vi "Create from SSH.vi"(8 "Error In":errorcluster, 11 "SSH":refnum<class "SSH.lvclass">) -> (0 "Error Out":errorcluster, 3 "Known Host":refnum<class "Known Host.lvclass">)   [LabVIEW 2018, in "Toolkit.lvlib" / "Known Host.lvclass"]
doc: "Creates a new Known Host object that represents a libssh2lv shared library Known Host struct. This VI must be called, or executed, before using any other Known Host-related VIs. This VI allocates memory within the libssh2lv shared library that must be explicitly deallocated, or freed, at the end of the application using the <B>Destroy</B> VI to avoid memory leaks or running Out-of-Memory (OOM) on a resource contrained system.\n\nA Known Host object represents the read-only data obtained about an entry in a known hosts file on the local host."
uses:
  Known Host.lvclass
  SSH/SSH.lvclass
  SSH/SSH.lvclass/SSH.ctl
  Known Host.lvclass/Known Host.ctl
  Toolkit.lvlib
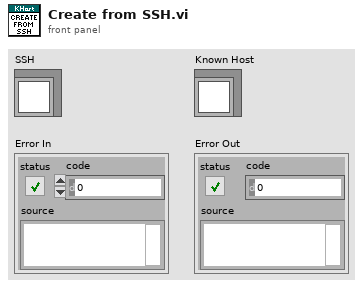
[diagram p1: front panel]
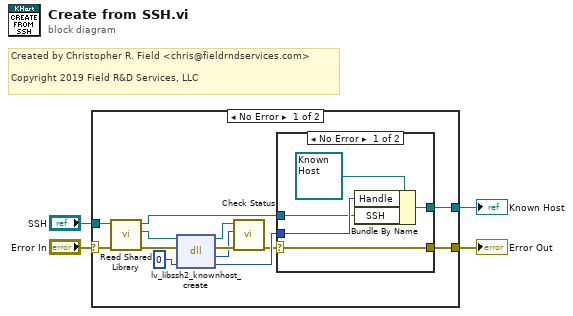
[diagram p0: block diagram]
diagram:
  # "Created by Christopher R. Field <chris@fieldrndservices.com>\n\nCopyright 2019 Field R&D Services, LLC"
  n1 = case shown="No Error" "Error In" {
    selector: "Error In" -> [w8 w24]
    tunnel: [w10 w24] -> w3
    tunnel: [w17 _] -> w2
    tunnel: "SSH" -> [w9 _]
    frame No Error {
      n2 = call "Read Shared Library.vi"("Error In"=w8, "SSH In"=w9) -> ("Error Out"=w7:errorcluster, "libssh2lv Shared Library"=w6:path, "SSH Out"=w5:refnum<class "SSH.lvclass">)  [unwired: 7 in]
      n3 = dll-call lib="D:/Users/cfield/Code/Field R&D Services/SSH/LV-LIBSSH2/LabVIEW/trunk/src/Toolkit/Support/lv-libssh2.*" fn="lv_libssh2_knownhost_create"(path in=w6, error in=w7, "handle"=u64 0) -> (path out=w13:path, error out=w14:errorcluster, "status"=w12:i32, "handle"=w15:u64)  [unwired: 1 in]
      n4 = call "Check Status.vi"("Error In"=w14, "Status"=w12, "libssh2lv Shared Library In"=w13) -> ("Error Out"=w11:errorcluster)  [unwired: 7 in, 1 out]
      n5 = case shown="No Error" w11 {
        selector: w11 -> [w20 w23]
        tunnel: [w22 _] -> w17
        tunnel: w15 -> [w21 _]
        tunnel: [w20 w23] -> w10
        tunnel: w5 -> [w18 _]
        frame No Error {
          n6 = Bundle By Name(cluster=refnum<class "Known Host.lvclass"> refnum ("Toolkit.lvlib:KnownHost.lvclass"), "Handle"=w21, "SSH"=w18) -> (w22:refnum<class "Known Host.lvclass">)
        }
        frame Error {
        }
      }
    }
    frame Error {
    }
  }
  "Error Out" <- w3
  "Known Host" <- w2
